vi "Set Speed.vi"(8 "error in (no error)":errorcluster, 10 "Speed (%)":dbl, 11 "Ismatech Settings In":T1={"VISA resource name"="", "Simulated?"=FALSE, "Pump Number"=1.0, "Reverse?"=FALSE} {"Pump Number" min=1.0 max=20.0 step=1.0}) -> (0 "error out":errorcluster, 1 "Connection Error":bool, 3 "Ismatech Settings Out":T1={"VISA resource name"="", "Simulated?"=FALSE, "Pump Number"=1.0, "Reverse?"=FALSE} {"Pump Number" min=1.0 max=20.0 step=1.0})   [LabVIEW 2021, in "Ismatec ISM 831C.lvlib"]
uses:
  Ismatec ISM 831C.lvlib
  Controls/Ismatech ISM831C Settings Cluster.ctl
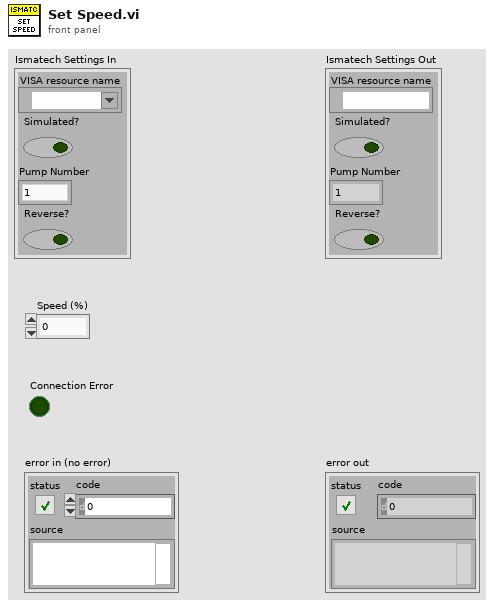
[diagram p1: front panel]
types:
  T1 = typedef "Ismatec ISM 831C.lvlib/Ismatech ISM831C Settings Cluster.ctl" = cluster{"VISA resource name":refnum<visa-resource-name>, "Simulated?":bool, "Pump Number":dbl, "Reverse?":bool}
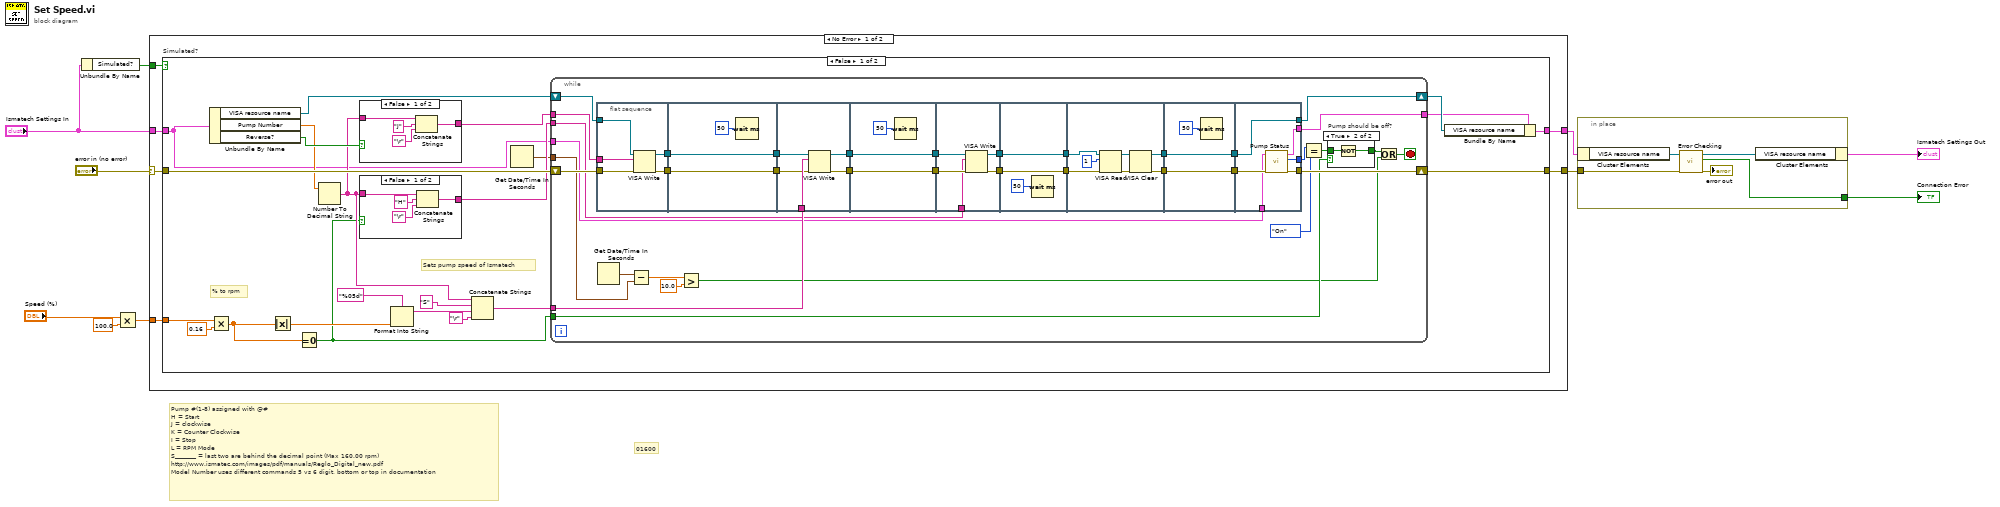
[diagram p0: block diagram]
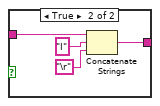
[diagram p3: hidden frame]
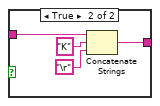
[diagram p4: hidden frame]
diagram:
  # "01600"
  # "Pump #(1-8) assigned with @#\nH = Start\nJ = clockwise\nK = Counter Clockwise\nI = Stop\nL = RPM Mode\nS_______ = last two are behind the decimal point (Max 160.00 rpm)\nhttp://www.ismatec.com/images/pdf/manuals/Reglo_Digital_new.pdf\nModel Number uses different commands 5 vs 6 digit, bottom or top in documentation"
  n1 = Unbundle By Name("Ismatech Settings In") -> ("Simulated?"=w8:bool)
  n2 = Multiply(x="Speed (%)", y=100.0) -> (x*y=w4:dbl)
  n3 = case shown="No Error" "error in (no error)" {
    selector: "error in (no error)" -> [w14 w138]
    tunnel: [w12 w137] -> w2
    tunnel: [w11 w138] -> w7
    tunnel: w4 -> [w13 _]
    tunnel: "Ismatech Settings In" -> [w16 w137]
    tunnel: w8 -> [w15 _]
    frame No Error {
      n4 = case "Simulated?" shown="False" w15 {
        tunnel: w13 -> [w33 _]
        tunnel: w16 -> [w21 w136]
        tunnel: [w39 w136] -> w12
        tunnel: w14 -> [w31 w135]
        tunnel: [w25 w135] -> w11
        frame False {
          # "% to rpm"
          # "Sets pump speed of Ismatech"
          n5 = Unbundle By Name(w21) -> ("VISA resource name"=w29:refnum<visa-resource-name>, "Pump Number"=w23:dbl, "Reverse?"=w26:bool)
          n6 = Multiply(x=w33, y=0.16) -> (x*y=w18:dbl)
          n7 = Absolute Value(x=w18) -> (abs(x)=w34:dbl)
          n8 = Equal To 0?(x=w18) -> (x = 0?=w17:bool)
          n9 = Number To Decimal String(number=w23) -> (decimal integer string=w22:string)  [unwired: 1 in]
          n10 = case shown="False" w26 {
            tunnel: w22 -> [w129 w134]
            tunnel: [w128 w132] -> w30
            frame False {
              n11 = Concatenate Strings(w129, "J" ("string"), "\r") -> (w128:string)
            }
            frame True {
              n12 = Concatenate Strings(w134, "K" ("string"), "\r") -> (w132:string)
            }
          }
          n13 = case shown="False" w17 {
            tunnel: [w120 w123] -> w27
            tunnel: w22 -> [w119 w124]
            frame False {
              n14 = Concatenate Strings(w119, "H", "\r") -> (w120:string)
            }
            frame True {
              n15 = Concatenate Strings(w124, "I", "\r") -> (w123:string)
            }
          }
          n16 = Format Into String(format string="%05d", w34) -> (resulting string=w36:string)  [unwired: 2 in, 1 out]
          n17 = Concatenate Strings(w22, "S" ("string"), w36, "\r") -> (w28:string)
          n18 = Get Date/Time In Seconds() -> (seconds since 1Jan1904=w19:timestamp)
          n19 = while {
            tunnel: w30 -> [w60]
            tunnel: w28 -> [w59]
            tunnel: w27 -> [w58]
            shift-right: [w57] -> w25
            shift-left: w31 -> [w61]
            shift-right: [w56] -> w24
            shift-left: w29 -> [w45]
            tunnel: w17 -> [w51]
            tunnel: w21 -> [w53]
            tunnel: [w52] -> w20
            tunnel: w19 -> [w43]
            stop <- w47 stop-if-true
            n20 = flat-sequence {
              tunnel: w61 -> [w83]
              tunnel: w60 -> [w82]
              tunnel: w45 -> [w81]
              tunnel: [w80] -> w75
              tunnel: [w79] -> w74
              tunnel: [w86] -> w73
              tunnel: w75 -> [w86]
              tunnel: w74 -> [w85]
              tunnel: [w85] -> w72
              tunnel: w59 -> [w91]
              tunnel: w73 -> [w90]
              tunnel: w72 -> [w89]
              tunnel: [w88] -> w71
              tunnel: [w87] -> w70
              tunnel: [w94] -> w69
              tunnel: w71 -> [w94]
              tunnel: w70 -> [w93]
              tunnel: [w93] -> w68
              tunnel: w69 -> [w97]
              tunnel: w68 -> [w96]
              tunnel: w58 -> [w95]
              tunnel: [w99] -> w67
              tunnel: [w98] -> w66
              tunnel: w67 -> [w102]
              tunnel: w66 -> [w101]
              tunnel: [w102] -> w65
              tunnel: [w101] -> w64
              tunnel: w65 -> [w109]
              tunnel: w64 -> [w107]
              tunnel: [w103] -> w63
              tunnel: [w105] -> w62
              tunnel: w63 -> [w112]
              tunnel: w62 -> [w111]
              tunnel: [w112] -> w55
              tunnel: [w111] -> w54
              tunnel: [w118] -> w56
              tunnel: [w116] -> w57
              tunnel: w55 -> [w117]
              tunnel: w54 -> [w118]
              tunnel: [w115] -> w42
              tunnel: w53 -> [w114]
              tunnel: [w113] -> w52
              frame #0 {
                n21 = VISA Write(VISA resource name=w81, write buffer=w82, error in (no error)=w83) -> (VISA resource name out=w80:refnum<visa-resource-name>, error out=w79:errorcluster)  [unwired: 1 out]
              }
              frame #1 {
                n22 = Wait (ms)(milliseconds to wait=u32 50) -> ()  [unwired: 1 out]
              }
              frame #2 {
                n23 = VISA Write(VISA resource name=w90, write buffer=w91, error in (no error)=w89) -> (VISA resource name out=w88:refnum<visa-resource-name>, error out=w87:errorcluster)  [unwired: 1 out]
              }
              frame #3 {
                n24 = Wait (ms)(milliseconds to wait=u32 50) -> ()  [unwired: 1 out]
              }
              frame #4 {
                n25 = VISA Write(VISA resource name=w97, write buffer=w95, error in (no error)=w96) -> (VISA resource name out=w98:refnum<visa-resource-name>, error out=w99:errorcluster)  [unwired: 1 out]
              }
              frame #5 {
                n26 = Wait (ms)(milliseconds to wait=u32 50) -> ()  [unwired: 1 out]
              }
              frame #6 {
                n27 = VISA Read(VISA resource name=w107, byte count=u32 1, error in (no error)=w109) -> (VISA resource name out=w106:refnum<visa-resource-name>, error out=w104:errorcluster)  [unwired: 2 out]
                n28 = VISA Clear(VISA resource name=w106, error in (no error)=w104) -> (VISA resource name out=w105:refnum<visa-resource-name>, error out=w103:errorcluster)
              }
              frame #7 {
                n29 = Wait (ms)(milliseconds to wait=u32 50) -> ()  [unwired: 1 out]
              }
              frame #8 {
                n30 = call "Pump Status.vi"("error in (no error)"=w117, "Ismatech Settings In"=w114) -> ("error out"=w116:errorcluster, "Pump On?"=w115:enum16{"Off", "On", "Not Initialized"}, "Ismatech Settings Out"=w113:T1)  [unwired: 6 in, 1 out]
              }
            }
            n31 = Get Date/Time In Seconds() -> (seconds since 1Jan1904=w44:timestamp)
            n32 = Subtract(x=w44, y=w43) -> (x-y=w50:dbl)
            n33 = Greater?(x=w50, y=10.0) -> (0:w46:bool)
            n34 = Equal?(x=w42, y=enum16{"Off", "On", "Not Initialized"}."On") -> (x = y?=w40:bool)
            n35 = case "Pump should be off?" shown="True" w51 {
              tunnel: w40 -> [w76 w78]
              tunnel: [w76 w77] -> w48
              frame False {
              }
              frame True {
                n36 = Not(x=w78) -> (.not. x?=w77:bool)
              }
            }
            n37 = Or(x=w48, y=w46) -> (x .or. y?=w47:bool)
          }
          n38 = Bundle By Name(cluster=w20, "VISA resource name"=w24) -> (w39:T1)
        }
        frame True {
        }
      }
    }
    frame Error {
    }
  }
  n39 = in-place {
    in-place-border: w7 -> [w143]
    in-place-border: [w141] -> w3
    n40 = in-place-cluster #1(w2) -> ("VISA resource name"=w140:refnum<visa-resource-name>)
    n41 = call "Error Checking.vi"("error in (no error)"=w143, "VISA resource name"=w140) -> ("error out"=→"error out":errorcluster, "Connection Error"=w141:bool, "VISA resource name"=w139:refnum<visa-resource-name>)  [unwired: 7 in]
    n42 = in-place-cluster #1("VISA resource name"=w139) -> (→"Ismatech Settings Out":T1)
  }
  "Connection Error" <- w3
